vi "Actor Core.vi"(8 "error in":errorcluster, 11 "MFC Actor.lvlib:MFC.lvclass":refnum<class "Valve.lvclass">) -> (0 "error out":errorcluster, 3 "Actor out":refnum<class "Actor.lvclass">)   [LabVIEW 2013, in "Valve.lvlib" / "Valve.lvclass"]
doc: "This is Actor Core.vi, the main message handling loop for Actors. An actor usually just sits in this loop and processes messages as they arrive. Any error returned by the message Do.vi call will stop the loop, with error code 43 as the canonical signal to stop with no error sent to caller. Descendants may override that in Handle Error.vi."
uses:
  Valve.lvclass
  PluginInterface/Actor Framework.lvlibp/Actor/Actor.lvclass
  Valve.lvclass/Valve.ctl
  PluginInterface/PluginInterface.lvlibp/PluginInterfaceClass/PluginInterface.lvclass
  PluginInterface/Actor Framework.lvlibp/Message Enqueuer/Message Priority.ctl
  Write Graph.vi
  Write Valve Position.vi
  Write Graph History.vi
  PluginInterface/PluginInterface.lvlibp/PluginInterfaceClass/Write VI Refnum.vi
  PluginInterface/Actor Framework.lvlibp/Message Enqueuer/Enqueue.vi
  Valve Messages/Initialize Msg/Initialize Msg.lvclass
  Valve Messages/Update Graphs Msg/Update Graphs Msg.lvclass
  Valve Messages/Update Setpoint Msg/Update Setpoint Msg.lvclass
  Valve Messages/Write MFC Msg/Write Valve Msg.lvclass
  PluginInterface/Actor Framework.lvlibp/Stop Msg/Stop Msg.lvclass
  PluginInterface/Actor Framework.lvlibp/Message Enqueuer/Message Enqueuer.lvclass
panel:
  in  "stop signal":bool
  in  "Valve Position":dbl(ring)=36.41913854673561 items=["0", "1", "2", "3", "4", "5", "6", "7"]
  in  "Graph History":dbl=300.0
  out "Graph 2":T1(graph) caption="Pump A"
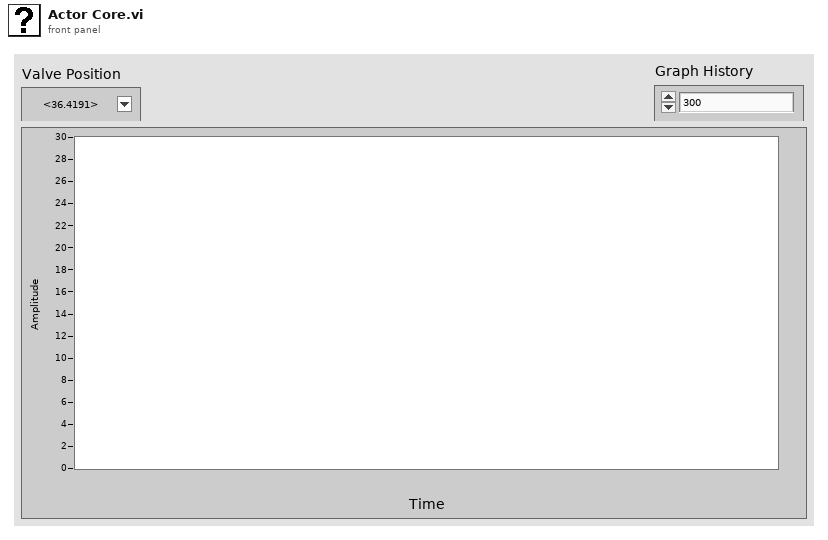
[diagram p1: front panel]
types:
  T1 = cluster{"output array":dbl[], "output array":dbl[]}
  T2 = typedef "Actor Framework.lvlibp/Message Enqueuer.lvclass/Message Priority.ctl" = enum16{"Low", "Normal", "High"}
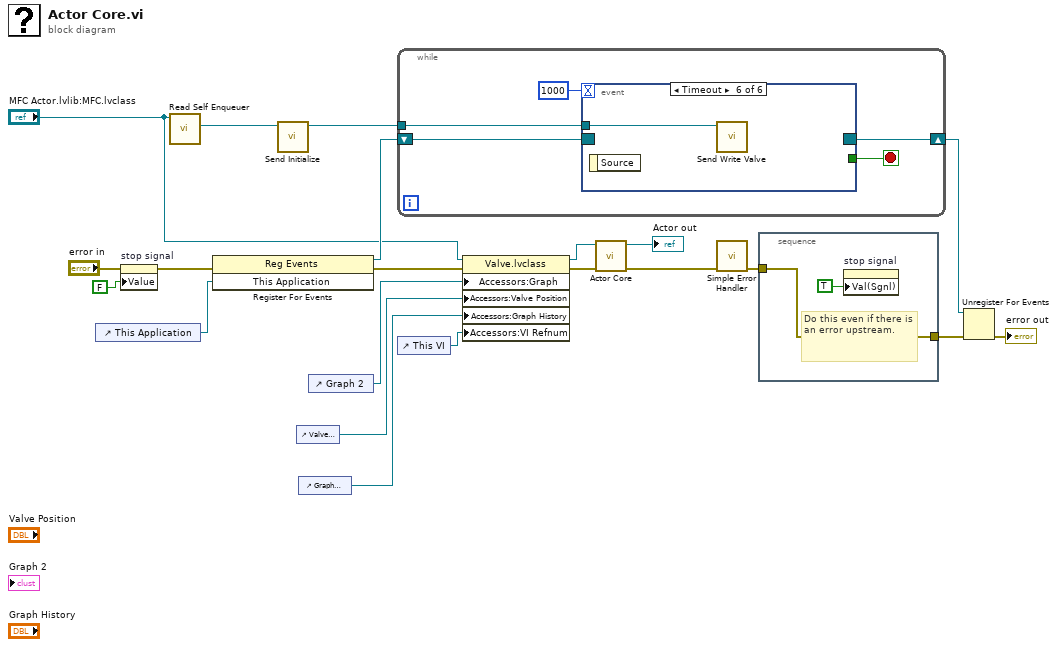
[diagram p0: block diagram]
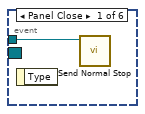
[diagram p2: hidden frame]
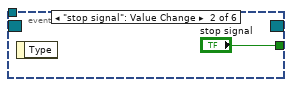
[diagram p3: hidden frame]
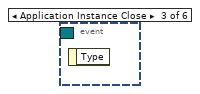
[diagram p4: hidden frame]
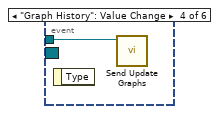
[diagram p5: hidden frame]
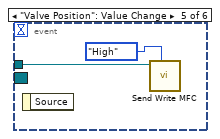
[diagram p6: hidden frame]
diagram:
  n1 = control-ref of="This Application"() -> (w14:refnum<vi>)
  n2 = property on="stop signal" class="Bool (strict)"(error in="error in", "Value"=FALSE ("stop")) -> (error out=w15:errorcluster)  [unwired: 1 in, 1 out]
  n3 = call "Read Self Enqueuer.vi"("Actor"="MFC Actor.lvlib:MFC.lvclass") -> ("Self Enqueuer"=w4:refnum<class "Message Enqueuer.lvclass">)  [unwired: 10 in]
  n4 = register-events(error in=w15, w14) -> (reference out=w18:refnum<event-registration>, error out=w2:errorcluster)  [unwired: 1 in]
  n5 = call "Send Initialize.vi"("Message Enqueuer"=w4) -> ("Message Enqueuer out"=w3:refnum<class "Message Enqueuer.lvclass">)  [unwired: 9 in, 1 out]
  n6 = control-ref of="Valve Position"() -> (w9:refnum<vi>)
  n7 = control-ref of="Graph History"() -> (w8:refnum<vi>)
  n8 = control-ref of="Graph 2"() -> (w5:refnum<vi>)
  n9 = while {
    tunnel: w3 -> [w26]
    shift-right: [w23] -> w17
    shift-left: w18 -> [w24]
    stop <- w25 stop-if-true
    n10 = event shown="[5] Timeout" {
      selector: w24 -> [_ _ _ _ _ _]
      dyn-events: [_ _ _ _ _ _] -> w23
      timeout: 1000 -> [_ _ _ _ _ _]
      tunnel: w26 -> [w27 _ _ w29 w31 w32]
      tunnel: [_ "stop signal" _ _ _ _] -> w25
      event Panel Close {
        n11 = event-data() -> ()  [unwired: 1 in, 1 out]
        n12 = call "Send Normal Stop.vi"("Message Enqueuer"=w27) -> ()  [unwired: 10 in, 1 out]
      }
      event "stop signal": Value Change {
        n13 = event-data() -> ()  [unwired: 1 in, 1 out]
      }
      event Application Instance Close {
        n14 = event-data() -> ()  [unwired: 1 in, 1 out]
      }
      event "Graph History": Value Change {
        n15 = event-data() -> ()  [unwired: 1 in, 1 out]
        n16 = call "Send Update Graphs.vi"("Message Enqueuer"=w29) -> ()  [unwired: 9 in, 2 out]
      }
      event "Valve Position": Value Change {
        n17 = event-data() -> ()  [unwired: 1 in, 1 out]
        n18 = call "Send Write MFC.vi"("Message Priority (Normal)"=Message_Priority."High", "Message Enqueuer"=w31) -> ()  [unwired: 8 in, 2 out]
      }
      event Timeout {
        n19 = event-data() -> ()  [unwired: 1 in, 1 out]
        n20 = call "Send Write Valve.vi"("Message Enqueuer"=w32) -> ()  [unwired: 9 in, 2 out]
      }
    }
  }
  n21 = control-ref of="This VI"() -> (w1:refnum<vi>)
  n22 = property class="Valve.lvclass"(reference="MFC Actor.lvlib:MFC.lvclass", error in=w2, "Accessors:Graph"=w5, "Accessors:Valve Position"=w9, "Accessors:Graph History"=w8, "Accessors:VI Refnum"=w1) -> (reference out=w7:refnum<class "Valve.lvclass">, error out=w10:errorcluster)
  n23 = call-parent "Actor Core.vi"("error in"=w10, "Actor in"=w7) -> ("error out"=w20:errorcluster, "Actor out"=→"Actor out":refnum<class "Actor.lvclass">)  [unwired: 8 in]
  n24 = call <vilib>:"Simple Error Handler.vi"("error in (no error)"=w20) -> ("error out"=w19:errorcluster)  [unwired: 4 in, 4 out]
  n25 = stacked-sequence {
    tunnel: [w33] -> w16
    tunnel: w19 -> [w33]
    frame #0 {
      # "Do this even if there is an error upstream."
      n26 = property on="stop signal" class="Bool (strict)"("Val(Sgnl)"=TRUE ("stop")) -> ()  [unwired: 2 in, 2 out]
    }
  }
  n27 = Unregister For Events(event registration refnum=w17, error in=w16) -> (error out=→"error out":errorcluster)
